vi "BeepWrapper.vi"() -> ()   [LabVIEW 2025]
panel:
  out "x = 0?":bool
  in  "x":dbl
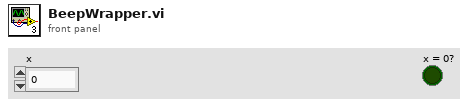
[diagram p1: front panel]
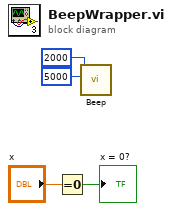
[diagram p0: block diagram]
diagram:
  n1 = Equal To 0?(x="x") -> (x = 0?=→"x = 0?":bool)
  n2 = call <vilib>:"Beep.vi"("duration (msec)"=u32 5000, "frequency (Hz)"=u32 2000) -> ()  [unwired: 10 in]
